vi "post.vi"(8 "error in (no error)":errorcluster, 10 "build_spec":T1, 11 "lv-builder-l3 in":refnum<class "lv-builder-l3.lvclass">) -> (0 "error out":errorcluster, 3 "lv-builder-l3 out":refnum<class "lv-builder-l3.lvclass">)   [LabVIEW 2015, in "lv-builder-l3.lvlib" / "lv-builder-l3.lvclass"]
uses:
  lv-builder-l3.lvclass
  lv-build/public/_controls/build_specification.ctl
  lv-build/public/_controls/build_type.ctl
  public/_controls/configuration.ctl
  lv-builder-l3.lvlib
  lv-build/lv-build.lvlib
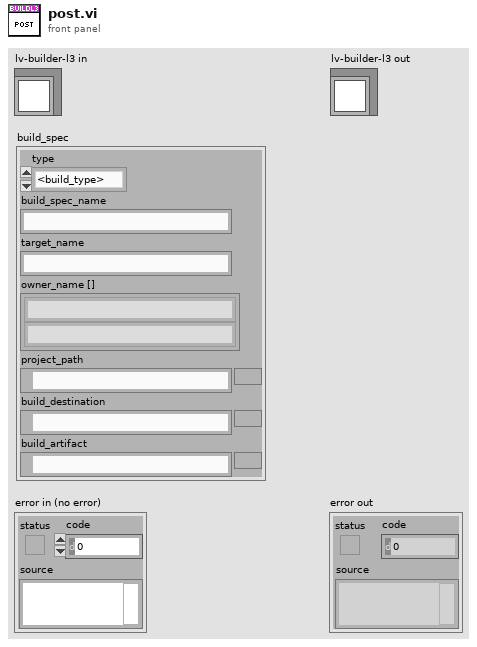
[diagram p1: front panel]
types:
  T1 = typedef "lv-build.lvlib/build_specification.ctl" = cluster{"type":T2, "build_spec_name":string, "target_name":string, "owner_name []":string[], "project_path":path, "build_destination":path, "build_artifact":path}
  T2 = typedef "lv-build.lvlib/build_type.ctl" = enum16{"<build_type>", "application_pc", "application_rt", "installer", "llb", "lvlibp", "zip", "fpga", "<null>"}
  T3 = typedef "lv-builder-l3.lvlib/configuration.ctl" = cluster{"l3_archive_file_path":string}
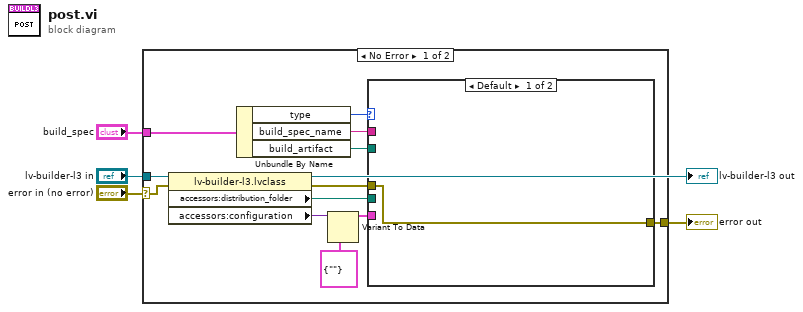
[diagram p0: block diagram]
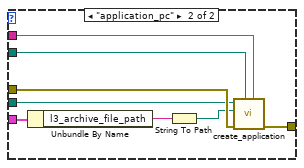
[diagram p2: hidden frame]
diagram:
  n1 = case shown="No Error" "error in (no error)" {
    selector: "error in (no error)" -> [w14 w26]
    tunnel: [w16 w26] -> w4
    tunnel: "build_spec" -> [w8 _]
    tunnel: "lv-builder-l3 in" -> [w15 _]
    frame No Error {
      n2 = property class="lv-builder-l3.lvclass"(reference=w15, error in=w14) -> (error out=w13:errorcluster, "accessors:distribution_folder"=w9:path, "accessors:configuration"=w10:variant)  [unwired: 1 out]
      n3 = Unbundle By Name(w8) -> ("type"=w7:T2, "build_spec_name"=w6:string, "build_artifact"=w5:path)
      n4 = Variant To Data(type=T3 {"l3_archive_file_path"=""} ("configuration"), Variant=w10) -> (data=w11:T3)  [unwired: 1 in, 1 out]
      n5 = case shown="Default" w7 {
        tunnel: [w17 w23] -> w16
        tunnel: w13 -> [w17 w25]
        tunnel: w11 -> [_ w24]
        tunnel: w9 -> [_ w20]
        tunnel: w6 -> [_ w22]
        tunnel: w5 -> [_ w21]
        frame Default {
        }
        frame "application_pc" {
          n6 = Unbundle By Name(w24) -> ("l3_archive_file_path"=w19:string)
          n7 = String To Path(string=w19) -> (path=w18:path)
          n8 = call "create_application.vi"("build_spec_name"=w22, "build_artifact"=w21, "error in (no error)"=w25, "l3_zip_file_path"=w18, "distribution_folder"=w20) -> ("error out"=w23:errorcluster)  [unwired: 6 in]
        }
      }
    }
    frame Error {
    }
  }
  "error out" <- w4
  "lv-builder-l3 out" <- "lv-builder-l3 in"
